vi "ATT Panel.vi"(8 "error in (no error)":errorcluster, 9 "ATT Configuration (\"\")":string, 10 "ATT Value In":T1={"Normalize"=TRUE, "Value (dB)"=0.0}, 11 "ATT Command":T2) -> (0 "error out":errorcluster, 1 "ATT Flat Output":string, 2 "ATT Value Out":T1={"Normalize"=TRUE, "Value (dB)"=0.0})   [LabVIEW 2011]
uses:
  tests/Attenuator/TypeDefs/Attenuator ATT Stimulus.ctl
  ATT Command.ctl
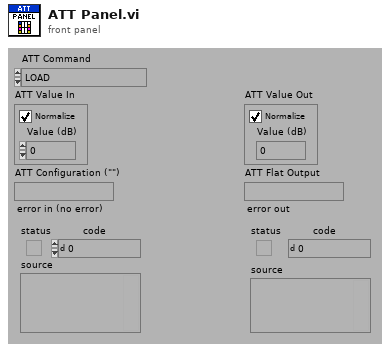
[diagram p1: front panel]
types:
  T1 = typedef "Attenuator ATT Stimulus.ctl" = cluster{"Normalize":bool, "Value (dB)":dbl}
  T2 = typedef "ATT Command.ctl" = enum16{"LOAD", "INITIALIZE", "PRESET", "SET STIMULUS", "GET STIMULUS", "GET CALIBRATION", "CALIBRATE", "GET INFO", "RELEASE", "UNLOAD"}
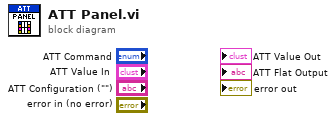
[diagram p0: block diagram]
diagram:
